vi "Path-gen.vi"(10 "Spreadsheet Name":string="%Y-%m-%d_%H-%M-%S.csv", 11 "Spreadsheet Path":path) -> (3 "appended path":path)   [LabVIEW 2025]
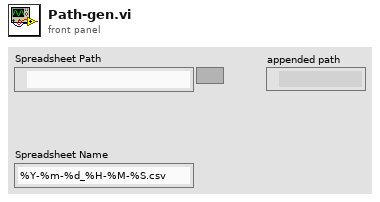
[diagram p1: front panel]
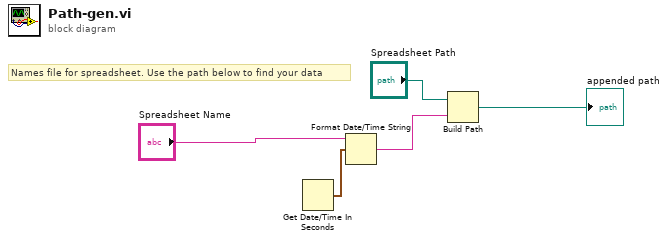
[diagram p0: block diagram]
diagram:
  # "Names file for spreadsheet. Use the path below to find your data"
  n1 = Get Date/Time In Seconds() -> (seconds since 1Jan1904=w2:timestamp)
  n2 = Format Date/Time String(time format string (%c)="Spreadsheet Name", seconds (now)=w2) -> (date/time string=w1:string)  [unwired: 1 in]
  n3 = Build Path(base path="Spreadsheet Path", name or relative path=w1) -> (appended path=→"appended path":path)
